vi "字符串操作函数（五）.vi"() -> ()   [LabVIEW 2010]
panel:
  out "字节数组":u8[](array[numeric])
  out "路径":path
  out "十进制数字符串":string
  out "小数字符串":string
  out "反转的字符串":string
  out "移位的字符串":string
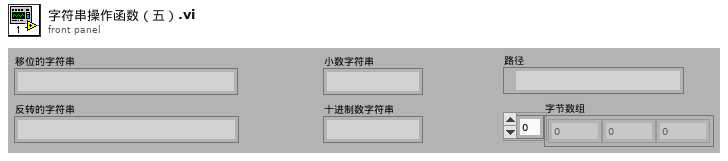
[diagram p1: front panel]
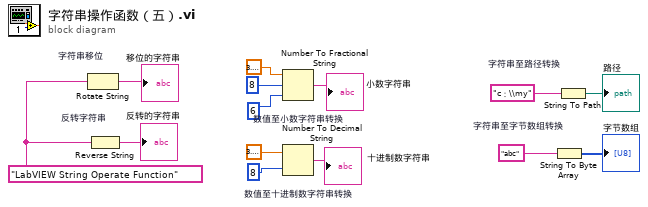
[diagram p0: block diagram]
diagram:
  w12 = "LabVIEW String Operate Function"
  n1 = Rotate String "字符串移位"(1:w12) -> (0:→"移位的字符串":string)
  n2 = Reverse String "反转字符串"(1:w12) -> (0:→"反转的字符串":string)
  n3 = Number To Fractional String "数值至小数字符串转换"(number=3.141592653589793, width (-)=8, precision (6)=6) -> (F-format string=→"小数字符串":string)  [unwired: 1 in]
  n4 = Number To Decimal String "数值至十进制数字符串转换"(number=3.141592653589793, width (-)=8) -> (decimal integer string=→"十进制数字符串":string)
  n5 = String To Byte Array "字符串至字节数组转换"(string="abc") -> (unsigned byte array=→"字节数组":u8[])
  n6 = String To Path "字符串至路径转换"(string="c：\\my") -> (path=→"路径":path)
